vi "Destroy Request Events.vi"(8 "error in":errorcluster) -> (0 "error out":errorcluster)   [LabVIEW 2021, in "MQTT Bridge.lvlib"]
doc: "Destroy the requests user events, even if there is an incoming error.\n\n<b>NOTE</b>: The contents of this VI are automatically generated and modified by the <b>Tools > DQMH Consortium > DQMH</b> utilities. Consider using those utilities instead of making your own modifications to this VI.\n_____\nBased on DQMH Dev Tools: Project Template 7.1.1.1528."
uses:
  MQTT Bridge.lvlib
panel:
  # "NOTE: The contents of this VI are automatically generated and modified by the Tools > DQMH Consortium > DQMH utilities. Consider using those utilities instead of making your own modifications to this VI."
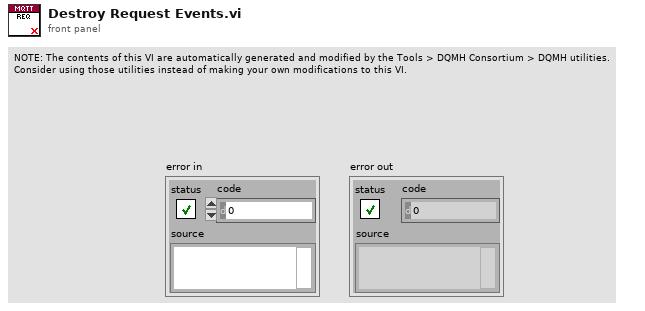
[diagram p1: front panel]
types:
  T1 = typedef "MQTT Bridge.lvlib/Request Events--cluster.ctl" = cluster{"Stop Module":refnum<user-event>, "Show Panel":refnum<user-event>, "Hide Panel":refnum<user-event>, "Show Diagram":refnum<user-event>, "Get Module Execution Status":refnum<user-event>, "Connect":refnum<user-event>, "Subscribe":refnum<user-event>, "Update Client Data":refnum<user-event>, "Disconnect":refnum<user-event>, "Check Connection":refnum<user-event>, "Ack Variable Write":refnum<user-event>, "Ack Run Start":refnum<user-event>, "Get Recipe":refnum<user-event>, "Run Finished":refnum<user-event>, "Test Result":refnum<user-event>}
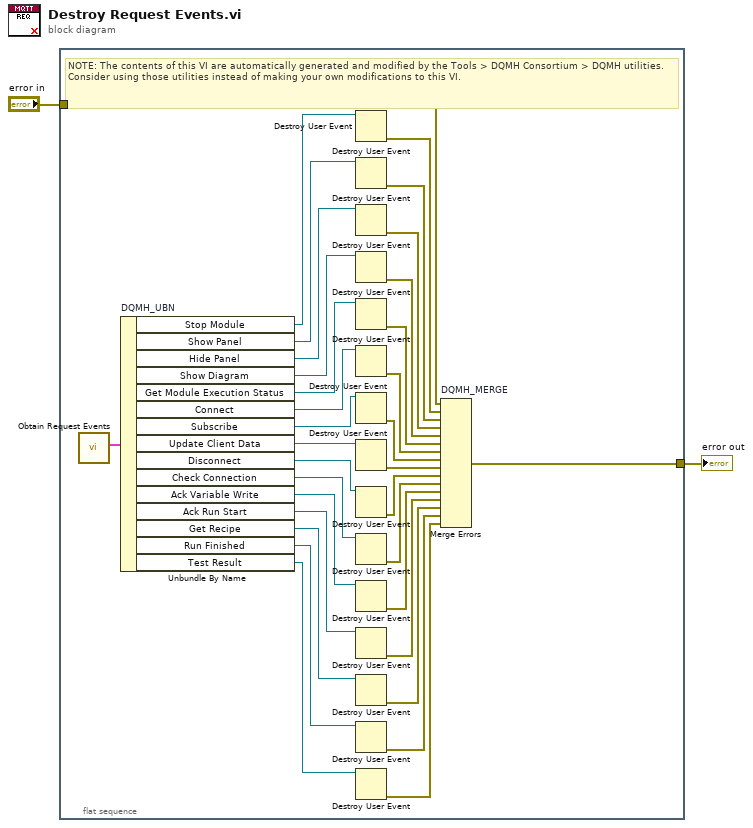
[diagram p0: block diagram]
diagram:
  n1 = flat-sequence {
    tunnel: [w34] -> w2
    tunnel: "error in" -> [w27]
    frame #0 {
      # "NOTE: The contents of this VI are automatically generated and modified by the Tools > DQMH Consortium > DQMH utilities. Consider using those utilities instead of making your own modifications to this VI."
      n2 = call "Obtain Request Events.vi"() -> ("MQTT Bridge Request Events"=w33:T1)  [unwired: 10 in, 1 out]
      n3 = Unbundle By Name "DQMH_UBN"(w33) -> ("Stop Module"=w32:refnum<user-event>, "Show Panel"=w29:refnum<user-event>, "Hide Panel"=w28:refnum<user-event>, "Show Diagram"=w25:refnum<user-event>, "Get Module Execution Status"=w23:refnum<user-event>, "Connect"=w21:refnum<user-event>, "Subscribe"=w19:refnum<user-event>, "Update Client Data"=w17:refnum<user-event>, "Disconnect"=w15:refnum<user-event>, "Check Connection"=w13:refnum<user-event>, "Ack Variable Write"=w11:refnum<user-event>, "Ack Run Start"=w9:refnum<user-event>, "Get Recipe"=w7:refnum<user-event>, "Run Finished"=w5:refnum<user-event>, "Test Result"=w3:refnum<user-event>)
      n4 = Destroy User Event(user event=w32) -> (error out=w35:errorcluster)  [unwired: 1 in]
      n5 = Destroy User Event(user event=w29) -> (error out=w31:errorcluster)  [unwired: 1 in]
      n6 = Destroy User Event(user event=w28) -> (error out=w30:errorcluster)  [unwired: 1 in]
      n7 = Destroy User Event(user event=w25) -> (error out=w26:errorcluster)  [unwired: 1 in]
      n8 = Destroy User Event(user event=w23) -> (error out=w24:errorcluster)  [unwired: 1 in]
      n9 = Destroy User Event(user event=w21) -> (error out=w22:errorcluster)  [unwired: 1 in]
      n10 = Destroy User Event(user event=w19) -> (error out=w20:errorcluster)  [unwired: 1 in]
      n11 = Destroy User Event(user event=w17) -> (error out=w18:errorcluster)  [unwired: 1 in]
      n12 = Destroy User Event(user event=w15) -> (error out=w16:errorcluster)  [unwired: 1 in]
      n13 = Destroy User Event(user event=w13) -> (error out=w14:errorcluster)  [unwired: 1 in]
      n14 = Destroy User Event(user event=w11) -> (error out=w12:errorcluster)  [unwired: 1 in]
      n15 = Destroy User Event(user event=w9) -> (error out=w10:errorcluster)  [unwired: 1 in]
      n16 = Destroy User Event(user event=w7) -> (error out=w8:errorcluster)  [unwired: 1 in]
      n17 = Destroy User Event(user event=w5) -> (error out=w6:errorcluster)  [unwired: 1 in]
      n18 = Destroy User Event(user event=w3) -> (error out=w4:errorcluster)  [unwired: 1 in]
      n19 = Merge Errors "DQMH_MERGE"(w27, w35, w31, w30, w26, w24, w22, w20, w18, w16, w14, w12, w10, w8, w6, w4) -> (w34:errorcluster)
    }
  }
  "error out" <- w2
